vi "Adjust temporary rotate and flip rectangle.vi"(11 "Pic in":picture) -> (2 "temp subset rect":cluster{i32, i32, "b-a":i32, "b-a":i32}, 3 "Pic out":picture, 4 "true subset rect":T1)   [LabVIEW 2021, in "lv_icon.lvlib"]
doc: "This function fixes coordinate changes in case the glyph is rotated or flipped."
uses:
  lv_icon.lvlib
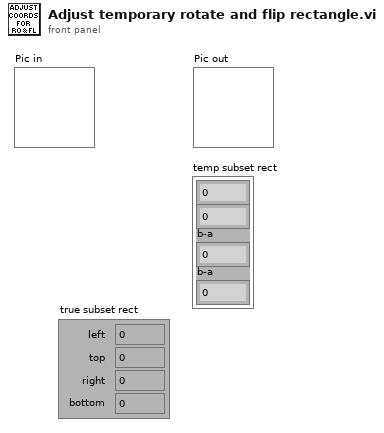
[diagram p1: front panel]
types:
  T1 = cluster{"left":i16, "top":i16, "right":i16, "bottom":i16}
  T2 = typedef "imagedata.ctl" = cluster{"image type":i32, "image depth":i32, "image":u8[], "mask":u8[], "colors":u32[], "Rectangle":cluster{"left":i16, "top":i16, "right":i16, "bottom":i16}}
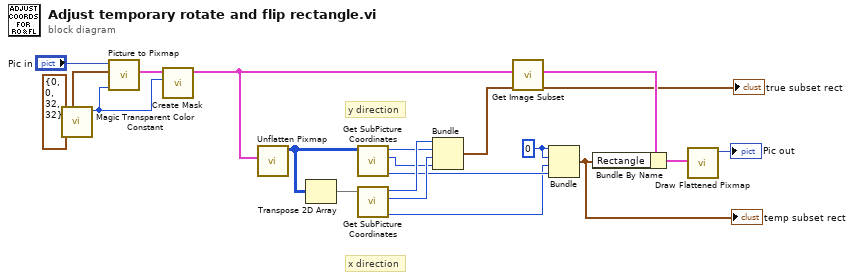
[diagram p0: block diagram]
diagram:
  w6 = 0
  # "y direction"
  # "x direction"
  n1 = call "Magic Transparent Color Constant.vi"() -> ("Magic transparent color constant"=w17:u32)  [unwired: 11 out]
  n2 = call <vilib>:"Picture to Pixmap.vi"("Background Color"=w17, "rect"=T1 {"left"=0, "top"=0, "right"=32, "bottom"=32}, "picture"="Pic in") -> ("image data"=w19:T2)  [unwired: 1 in, 7 out]
  n3 = call <vilib>:"Create Mask.vi"("Mask Color (Black)"=w17, "image data"=w19) -> ("image data"=w16:T2)  [unwired: 2 in, 7 out]
  n4 = call <vilib>:"Unflatten Pixmap.vi"("image data"=w16) -> ("24-bit pixmap"=w15:u32[][])  [unwired: 10 out]
  n5 = Transpose 2D Array(2D array=w15) -> (transposed array=w14:u32[][])
  n6 = call "Get SubPicture Coordinates.vi"("24-bit pixmap"=w15) -> ("b-a"=w8:i32, "b"=w10:i32, "a"=w12:i32)  [unwired: 8 out]
  n7 = call "Get SubPicture Coordinates.vi"("24-bit pixmap"=w14) -> ("b-a"=w7:i32, "b"=w11:i32, "a"=w13:i32)  [unwired: 8 out]
  n8 = Bundle("a"=w13, "a"=w12, "b"=w11, "b"=w10) -> (w9:cluster{"a":i32, "a":i32, "b":i32, "b":i32})  [unwired: 1 out]
  n9 = call <vilib>:"Get Image Subset.vi"("subset rect"=w9, "image data"=w16) -> ("true subset rect"=→"true subset rect":T1, "image subset"=w5:T2)  [unwired: 4 out]
  n10 = Bundle(w6, w6, "b-a"=w7, "b-a"=w8) -> (w4:cluster{i32, i32, "b-a":i32, "b-a":i32})  [unwired: 1 out]
  "temp subset rect" <- w4
  n11 = Bundle By Name(cluster=w5, "Rectangle"=w4) -> (w3:T2)
  n12 = call <vilib>:"Draw Flattened Pixmap.vi"("image data"=w3) -> ("new picture"=→"Pic out":picture)  [unwired: 1 in, 7 out]
